vi "Read.vi"(0 "channel":T1, 1 "timeout in ms (0)":i32) -> (2 "missed":i32, 3 "element":string)   [LabVIEW 2020, in "Tag-str.lvlib"]
doc: "Reads a value from a Tag channel."
uses:
  <extravilib>/ChannelInstances/Tag-str.lvlib
  <extravilib>/ChannelInstances/Tag-str/))Channel.ctl
panel:
  # "number of values missed\n(-1 means element is stale)"
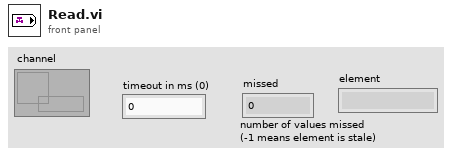
[diagram p1: front panel]
types:
  T1 = typedef "Tag-str.lvlib/))Channel.ctl" = refnum<queue>
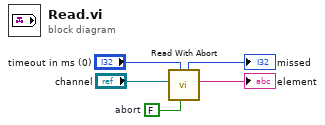
[diagram p0: block diagram]
diagram:
  w1 = FALSE  # abort
  n1 = call <extravilib>:"Read With Abort.vi"("abort"=w1, "timeout in ms (0)"="timeout in ms (0)", "channel"="channel") -> ("element"=→"element":string, "missed"=→"missed":i32)  [unwired: 6 in, 1 out]
